vi "Delete Tree.vi"(8 "error in (no error)":errorcluster, 11 "UA Server in":refnum<class "UA Server.lvclass">) -> (0 "error out":errorcluster)   [LabVIEW 2017, in "opcua.lvlib" / "Browser Core.lvlib" / "UA Server.lvclass"]
doc: "Use this as the destructor for the tree object"
uses:
  UA Server.lvclass
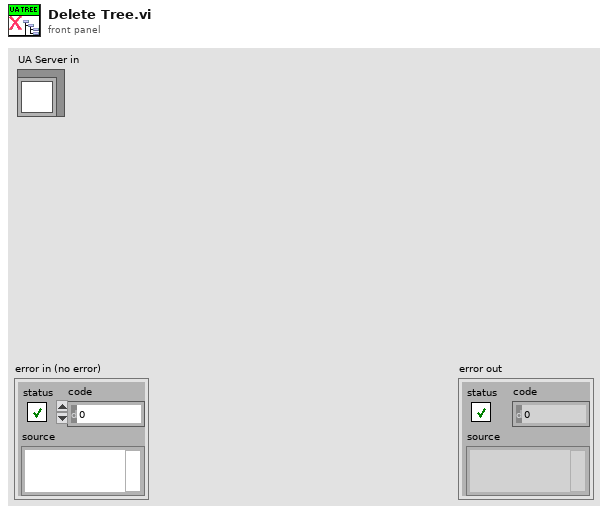
[diagram p1: front panel]
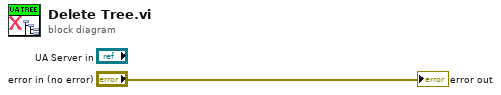
[diagram p0: block diagram]
diagram:
  "error out" <- "error in (no error)"
